vi "NIPKG to Package URL.vi"(11 "package attributes":T1={"Package Name"="", "Display name"="", "Version"="", "Display version"="", "Synopsis"="", "Description"="", "Maintainer"="", "Maintainer email address"="", "Category"="", "Homepage"="", "Release notes"="", "Depends"=[], "Recommends"=[], "Suggests"=[], "Conflicts"=[], "Provides"=[], "Replaces"=[], "Supplements"=[], "Enhances"=[], "Product"=FALSE, "User visible"=FALSE, "Installed size (KB)"=0, "Package filesize (bytes)"=0, "Architecture"="", "Agent"="file", "MD5Checksum"=""}) -> (3 "NIPKG Package URL":string)   [LabVIEW 2017, in "NIPKG SBOM Support.lvlib"]
doc: "Converts NIPKG information to a pURL package URL"
uses:
  NIPKG SBOM Support.lvlib
  <vilib>/National Instruments/NIPM API (Beta)/_support/package attributes.ctl
  <vilib>/wsapi/NI_WebServices.lvlib
  <vilib>/National Instruments/NIPM API (Beta)/NIPM_API.lvlib
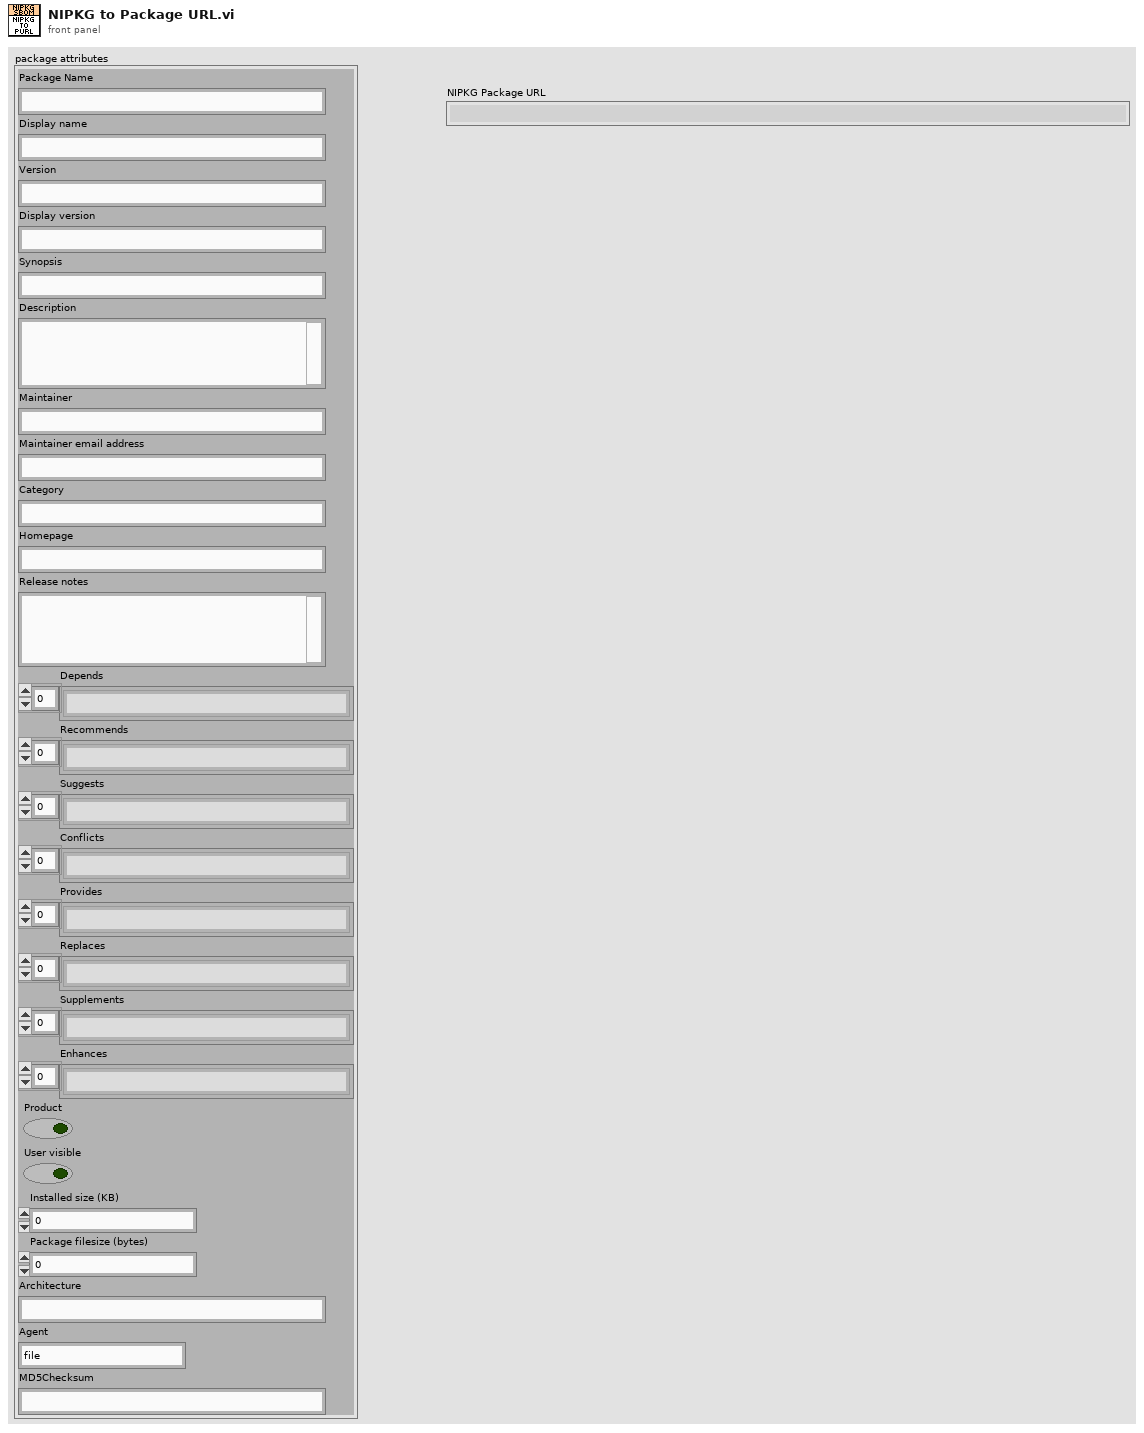
[diagram p1: front panel]
types:
  T1 = typedef "NIPM_API.lvlib/package attributes.ctl" = cluster{"Package Name":string, "Display name":string, "Version":string, "Display version":string, "Synopsis":string, "Description":string, "Maintainer":string, "Maintainer email address":string, "Category":string, "Homepage":string, "Release notes":string, "Depends":string[], "Recommends":string[], "Suggests":string[], "Conflicts":string[], "Provides":string[], "Replaces":string[], "Supplements":string[], "Enhances":string[], "Product":bool, "User visible":bool, "Installed size (KB)":u64, "Package filesize (bytes)":u64, "Architecture":string, "Agent":string, "MD5Checksum":string}
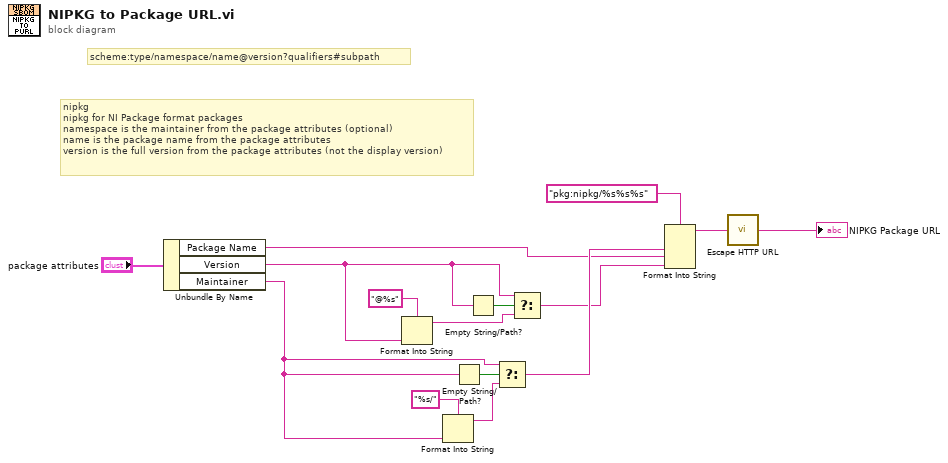
[diagram p0: block diagram]
diagram:
  # "nipkg\nnipkg for NI Package format packages\nnamespace is the maintainer from the package attributes (optional)\nname is the package name from the package attributes\nversion is the full version from the package attributes (not the display version)"
  # "scheme:type/namespace/name@version?qualifiers#subpath"
  n1 = Unbundle By Name("package attributes") -> ("Package Name"=w1:string, "Version"=w3:string, "Maintainer"=w10:string)
  n2 = Format Into String(format string="@%s", w3) -> (resulting string=w6:string)  [unwired: 2 in, 1 out]
  n3 = Format Into String(format string="%s/", w10) -> (resulting string=w9:string)  [unwired: 2 in, 1 out]
  n4 = Empty String/Path?(string/path=w10) -> (empty?=w12:bool)
  n5 = Empty String/Path?(string/path=w3) -> (empty?=w4:bool)
  n6 = Select(t=w10, s=w12, f=w9) -> (s? t:f=w11:string)
  n7 = Select(t=w3, s=w4, f=w6) -> (s? t:f=w5:string)
  n8 = Format Into String(format string="pkg:nipkg/%s%s%s", w11, w1, w5) -> (resulting string=w14:string)  [unwired: 2 in, 1 out]
  n9 = call <vilib>:"Escape HTTP URL.vi"("unescaped string in"=w14) -> ("escaped string out"=→"NIPKG Package URL":string)
